vi "模拟输入_电流_软件按需单点.vi"() -> ()   [LabVIEW 2013]
doc: "This example demonstrates how to measure voltage using a software timer."
uses:
  <userlib>/ArtDAQ/_SubVI/ArtDAQ_CreateAICurrentChan.vi
  <userlib>/ArtDAQ/_SubVI/ArtDAQ_Read Analog DBL NChan 1Samp.vi
panel:
  in  "外部分流电阻值":dbl=249.0 format="%.2f"
  in  "分流电阻位置":i32(ring)=-1 items=["默认"=-1, "内部"=10200, "外部"=10167]
  out "数据":dbl[](array[numeric])
  in  "定时 (ms)":u32=100
  in  "Stop":bool
  in  "最小值(A)":dbl format="%#_13g"
  in  "最大值(V)":dbl=0.02 format="%#_13g"
  in  "物理通道":string(combo)="Dev1/ai0"
  out "错误":errorcluster
  # "通道属性"
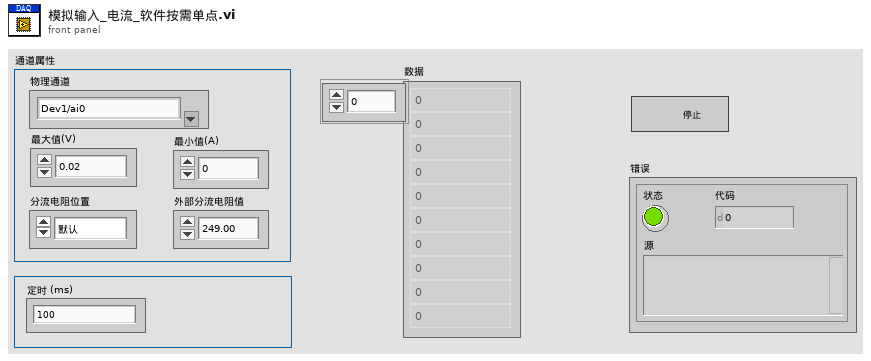
[diagram p1: front panel]
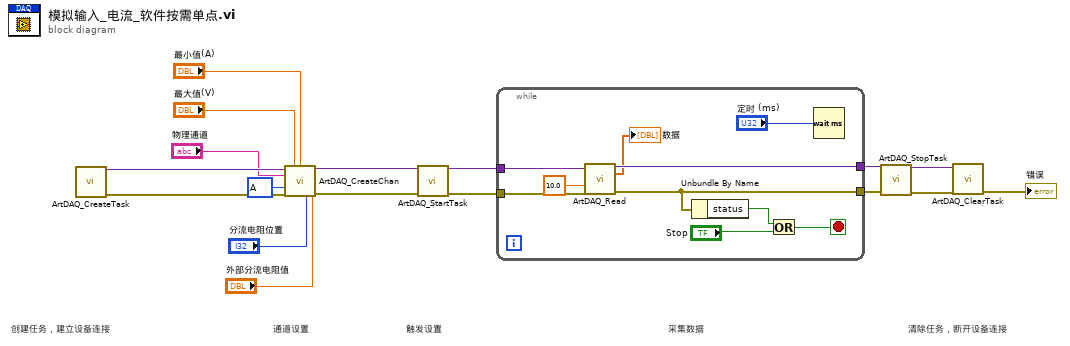
[diagram p0: block diagram]
diagram:
  w1 = 10342 items=["默认"=-1, "A"=10342] ("单位")
  # "清除任务，断开设备连接"
  # "采集数据"
  # "触发设置"
  # "通道设置"
  # "创建任务，建立设备连接"
  n1 = call <userlib>:"ArtDAQ_CreateTask.vi"() -> ("任务句柄"=w11:variant, "错误输出"=w17:errorcluster)  [unwired: 14 in]
  n2 = call-poly <userlib>:"ArtDAQ_CreateChan.vi"("任务句柄"=w11, "最大值"="最大值(V)", "最小值"="最小值(A)", "物理通道"="物理通道", "外部分流电阻值"="外部分流电阻值", "单位"=w1, "错误输入"=w17, "分流电阻位置"="分流电阻位置") -> ("任务句柄"=w5:variant, "错误输出"=w4:errorcluster)  [unwired: 6 in]
  n3 = call <userlib>:"ArtDAQ_StartTask.vi"("任务句柄"=w5, "错误输入"=w4) -> ("任务句柄"=w13:variant, "错误输出"=w12:errorcluster)  [unwired: 12 in]
  n4 = while {
    tunnel: w13 -> [w27]
    tunnel: w12 -> [w26]
    tunnel: [w24] -> w10
    tunnel: [w23] -> w9
    stop <- w21 stop-if-true
    n5 = call-poly <userlib>:"ArtDAQ_Read.vi"("任务句柄"=w27, "超时s"=10.0 ("Timeout"), "错误输入"=w26) -> ("任务句柄"=w24:variant, "数据"=→"数据":dbl[], "错误输出"=w23:errorcluster)  [unwired: 10 in]
    n6 = Unbundle By Name(w23) -> ("status"=w22:bool)
    n7 = Or(x=w22, y="Stop") -> (x .or. y?=w21:bool)
    n8 = Wait (ms)(milliseconds to wait="定时 (ms)") -> ()  [unwired: 1 out]
  }
  n9 = call <userlib>:"ArtDAQ_StopTask.vi"("任务句柄"=w10, "错误输入"=w9) -> ("任务句柄"=w8:variant, "错误输出"=w7:errorcluster)  [unwired: 12 in]
  n10 = call <userlib>:"ArtDAQ_ClearTask.vi"("任务句柄"=w8, "错误输入"=w7) -> ("错误输出"=→"错误":errorcluster)  [unwired: 13 in]
